vi "Hold Data.vi"(0 "VISA resource name":refnum<visa-resource-name>, 5 "Hold (F: OFF)":bool, 11 "error in (no error)":errorcluster) -> (4 "VISA resource name out":refnum<visa-resource-name>, 15 "error out":errorcluster)   [LabVIEW 2010, in "Yokogawa WT200 Series.lvlib"]
doc: "This VI sends the display value hold command to the WT200 Series."
uses:
  G:/Engineering/Retail/LabV/instr.lib/Yokogawa WT200 Series/Yokogawa WT200 Series.lvlib
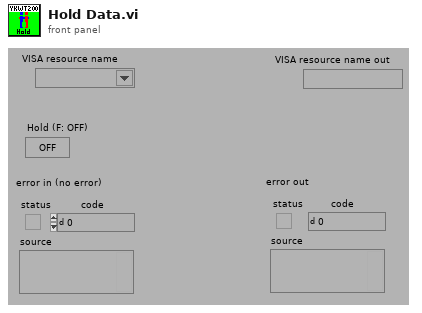
[diagram p1: front panel]
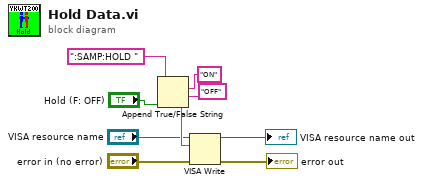
[diagram p0: block diagram]
diagram:
  n1 = Append True/False String(1:"Hold (F: OFF)", 2:"OFF", 3:"ON", 4:":SAMP:HOLD ") -> (0:w9:string)
  n2 = VISA Write(VISA resource name="VISA resource name", write buffer=w9, error in (no error)="error in (no error)") -> (VISA resource name out=→"VISA resource name out":refnum<visa-resource-name>, error out=→"error out":errorcluster)  [unwired: 1 out]
